vi "U32 to U64.vi"(1 "U32":u32) -> (0 "U64 cast as DBL":dbl)   [LabVIEW 2017]
panel:
  # "LVHDF5 Toolkit\nCopyright (c) 2005-2013 by Jason D. Sommerville\nCopyright (c) 2014 by UPVI, LLC.\n\nThis use and distribution of this file is governed by the terms found in \nLICENSE.txt distributed with this toolkit and installed at\n <user.lib>\\_lvhdf5\\LICENSE.txt"
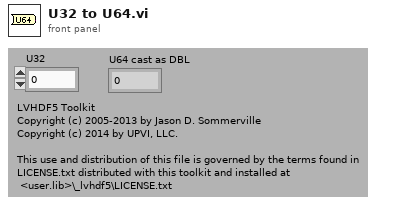
[diagram p1: front panel]
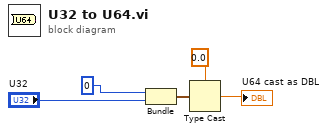
[diagram p0: block diagram]
diagram:
  n1 = Bundle(u32 0, "U32"="U32") -> (w4:cluster{u32, "U32":u32})  [unwired: 1 in]
  n2 = Type Cast(type=0.0, x=w4) -> (*(type *) &x=→"U64 cast as DBL":dbl)
